vi "VMI_move_wait_PI.vi"(3 "Scan?":bool, 4 "SetV?":bool, 5 "Stage Position 2":refnum<vi>, 6 "Move and Wait?":bool, 7 "Delay Cluster":T1={"System no."=0, "Identification"="", "Device ID out"=0, "Postion / mm"=[], "SN out"="", "Movement Range"=[], "Conn. Axes"=[], "Target Position / mm"=50.0, "Velocity / mm s^-1"=0.15, "Set-up"=FALSE, "Moving"=FALSE, "Step Size / mm "=0.15, "Stage Number"=0, "Polling Time /ms"=0, "Delay Scan?"=FALSE, "Accurate Scan"=FALSE, "CmdMovDelay"=FALSE, "CmdStopDelay"=FALSE, "Delay List"=[["Number", "Target / mm", "Relative Integration Time"]], "Scan Start /mm"=50.0, "Scan End / mm"=80.0, "Scan Velocity / mm s^-1"=0.15, "Delay Scan Time / s"=30.0}, 8 "Error In":errorcluster, 10 "Stop ref":refnum<vi>, 11 "Postion / mm":refnum<vi>) -> (0 "error out":errorcluster)   [LabVIEW 2020]
uses:
  Type defs/PI_delay_settings_alt.ctl
panel:
  out "Stage Position":dbl=50.0
  in  "Stop Button":bool
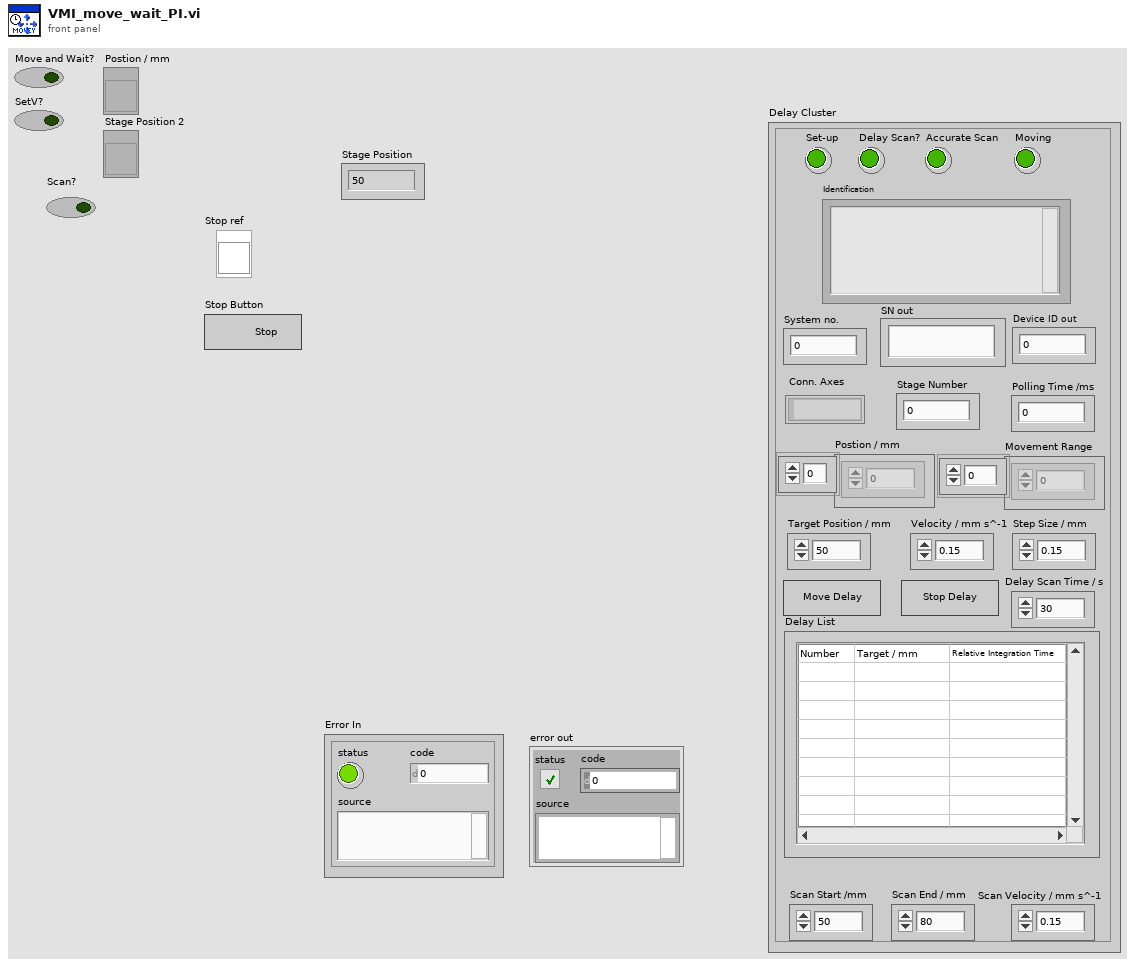
[diagram p1: front panel]
types:
  T1 = typedef "PI_delay_settings_alt.ctl" = cluster{"System no.":i32, "Identification":string, "Device ID out":i32, "Postion / mm":dbl[], "SN out":string, "Movement Range":dbl[], "Conn. Axes":string[], "Target Position / mm":dbl, "Velocity / mm s^-1":dbl, "Set-up":bool, "Moving":bool, "Step Size / mm ":dbl, "Stage Number":i32, "Polling Time /ms":i32, "Delay Scan?":bool, "Accurate Scan":bool, "CmdMovDelay":bool, "CmdStopDelay":bool, "Delay List":string[][], "Scan Start /mm":dbl, "Scan End / mm":dbl, "Scan Velocity / mm s^-1":dbl, "Delay Scan Time / s":dbl}
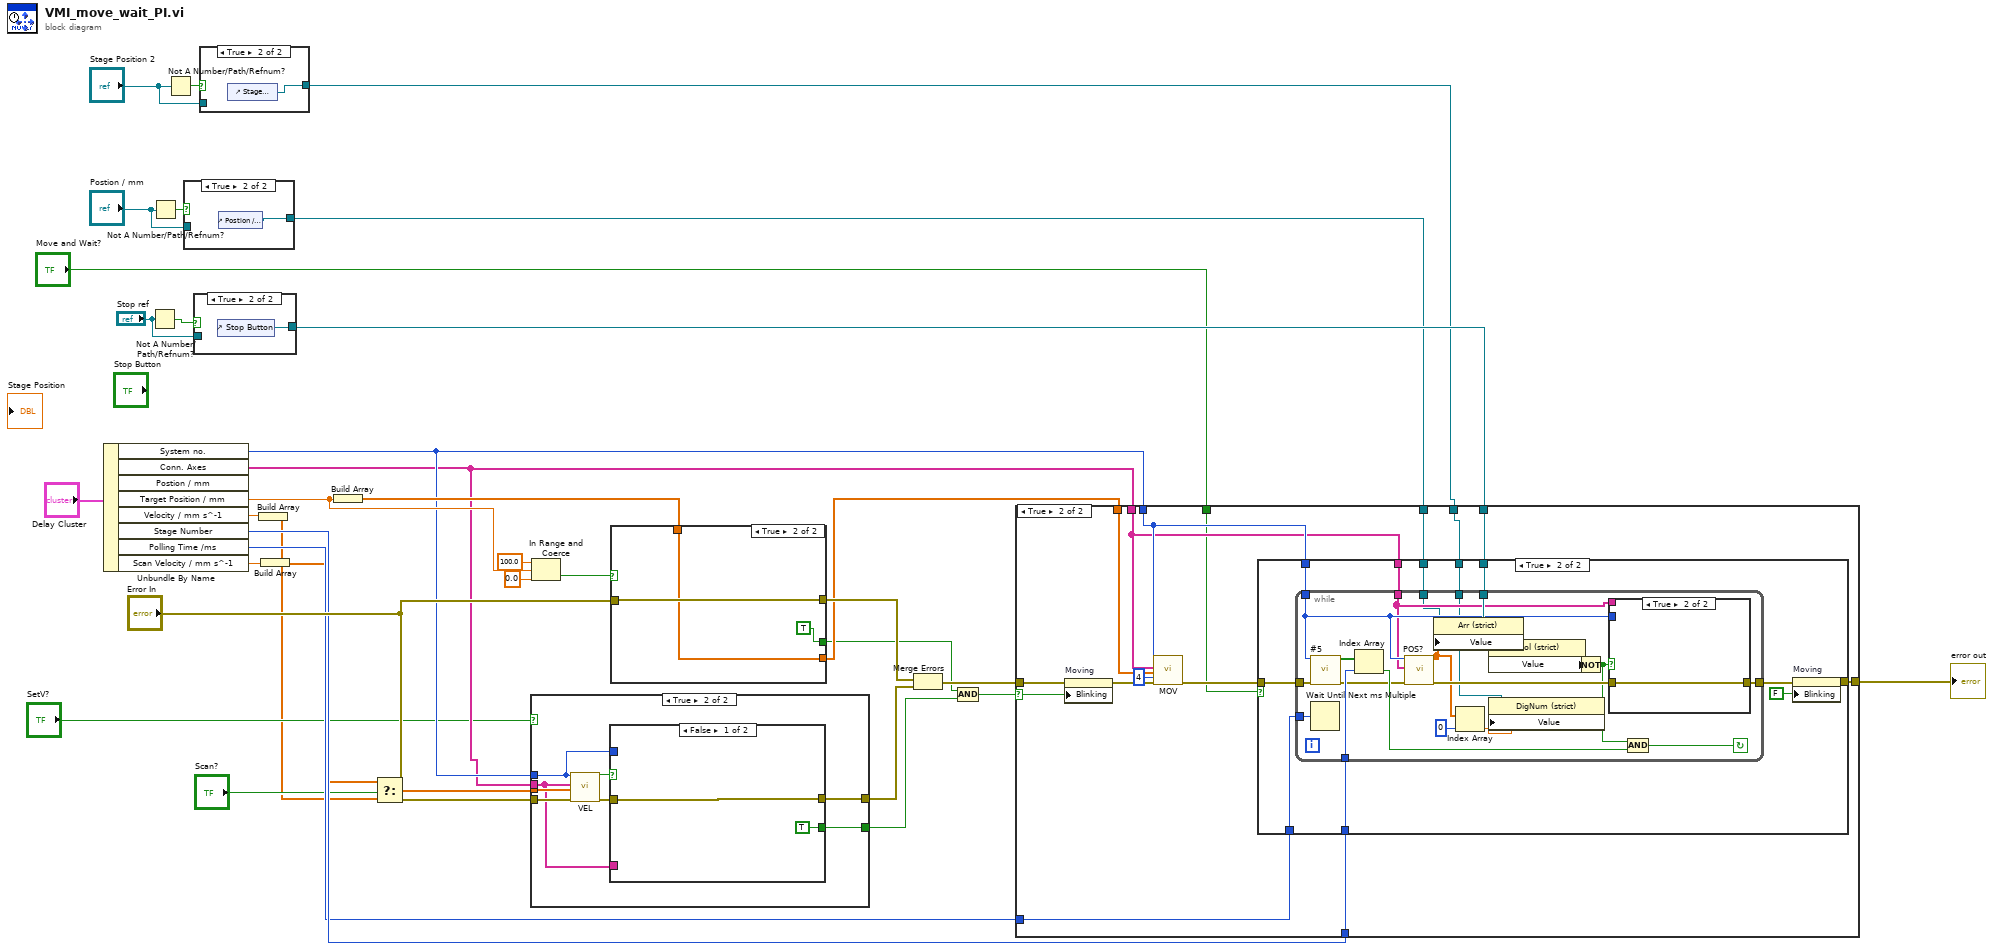
[diagram p0: block diagram]
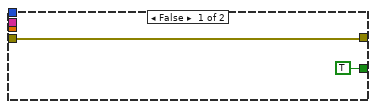
[diagram p3: hidden frame]
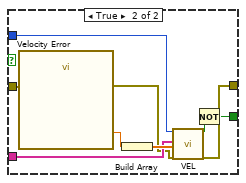
[diagram p4: hidden frame]
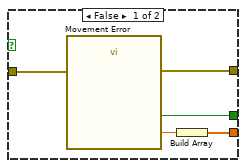
[diagram p7: hidden frame]
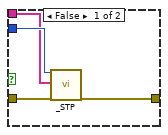
[diagram p10: hidden frame]
diagram:
  n1 = Unbundle By Name("Delay Cluster") -> ("System no."=w18:i32, "Conn. Axes"=w17:string[], "Target Position / mm"=w27:dbl, "Velocity / mm s^-1"=w35:dbl, "Stage Number"=w14:i32, "Polling Time /ms"=w13:i32, "Scan Velocity / mm s^-1"=w8:dbl)  [unwired: 1 out]
  n2 = Not A Number/Path/Refnum?(number/path/refnum="Stop ref") -> (NaN/Path/Refnum?=w21:bool)
  n3 = Not A Number/Path/Refnum?(number/path/refnum="Postion / mm") -> (NaN/Path/Refnum?=w15:bool)
  n4 = Not A Number/Path/Refnum?(number/path/refnum="Stage Position 2") -> (NaN/Path/Refnum?=w3:bool)
  n5 = case shown="True" w15 {
    tunnel: "Postion / mm" -> [w37 _]
    tunnel: [w37 w38] -> w10
    frame False {
    }
    frame True {
      n6 = control-ref of="Postion / mm"() -> (w38:refnum<vi>)
    }
  }
  n7 = case shown="True" w21 {
    tunnel: [w39 w40] -> w19
    tunnel: "Stop ref" -> [w39 _]
    frame False {
    }
    frame True {
      n8 = control-ref of="Stop Button"() -> (w40:refnum<vi>)
    }
  }
  n9 = case shown="True" w3 {
    tunnel: "Stage Position 2" -> [w41 _]
    tunnel: [w41 w42] -> w1
    frame False {
    }
    frame True {
      n10 = control-ref of="Stage Position"() -> (w42:refnum<vi>)
    }
  }
  n11 = Build Array(w35) -> (w5:dbl[])
  n12 = Build Array(w8) -> (w6:dbl[])
  n13 = Build Array(w27) -> (w30:dbl[])
  n14 = Select(t=w6, s="Scan?", f=w5) -> (s? t:f=w4:dbl[])
  n15 = case shown="True" "SetV?" {
    tunnel: w4 -> [_ w52]
    tunnel: "Error In" -> [w44 w49]
    tunnel: [w44 w48] -> w32
    tunnel: [TRUE ("OK") w47] -> w24
    tunnel: w18 -> [_ w46]
    tunnel: w17 -> [_ w45]
    frame False {
    }
    frame True {
      n16 = call "VEL.vi"("System no."=w46, "Axes to set"=w45, "Velocity values"=w52, "error in"=w49) -> ("Controller error"=w51:bool, "error out"=w50:errorcluster)  [unwired: 2 in, 12 out]
      n17 = case shown="False" w51 {
        tunnel: w50 -> [w54 w63]
        tunnel: [w54 w57] -> w48
        tunnel: [TRUE ("OK") w55] -> w47
        tunnel: w46 -> [_ w60]
        tunnel: w45 -> [_ w59]
        frame False {
        }
        frame True {
          n18 = call "Velocity Error"("error in (no error)"=w63) -> ("Velocity"=w62:dbl, "error out"=w58:errorcluster)  [unwired: 16 in, 1 out]
          n19 = Build Array(w62) -> (w61:dbl[])
          n20 = call "VEL.vi"("System no."=w60, "Axes to set"=w59, "Velocity values"=w61, "error in"=w58) -> ("Controller error"=w56:bool, "error out"=w57:errorcluster)  [unwired: 2 in, 12 out]
          n21 = Not(x=w56) -> (.not. x?=w55:bool)
        }
      }
    }
  }
  n22 = In Range and Coerce(upper limit=100.0, x=w27, lower limit=0.0) -> (In Range?=w25:bool)  [unwired: 1 out]
  n23 = case shown="True" w25 {
    tunnel: "Error In" -> [w68 w71]
    tunnel: [w67 w71] -> w33
    tunnel: [w66 TRUE ("OK")] -> w22
    tunnel: [w64 w69] -> w29
    tunnel: w30 -> [_ w69]
    frame False {
      n24 = call "Movement Error"("error in (no error)"=w68) -> ("Target"=w65:dbl, "OK"=w66:bool, "error out"=w67:errorcluster)  [unwired: 16 in]
      n25 = Build Array(w65) -> (w64:dbl[])
    }
    frame True {
    }
  }
  n26 = Merge Errors(w33, w32) -> (w31:errorcluster)
  n27 = And(x=w22, y=w24) -> (x .and. y?=w23:bool)
  n28 = case shown="True" w23 {
    selector: w23 -> [_ w84]
    tunnel: w29 -> [_ w87]
    tunnel: w18 -> [_ w80]
    tunnel: w17 -> [_ w78]
    tunnel: w31 -> [w72 w85]
    tunnel: [w72 w82] -> w16
    tunnel: w14 -> [_ w79]
    tunnel: w19 -> [_ w77]
    tunnel: w13 -> [_ w76]
    tunnel: "Move and Wait?" -> [_ w75]
    tunnel: w10 -> [_ w74]
    tunnel: w1 -> [_ w73]
    frame False {
    }
    frame True {
      n29 = property on="Moving" class="Bool (strict)"(error in=w85, "Blinking"=w84) -> (error out=w83:errorcluster)  [unwired: 1 in, 1 out]
      n30 = call "MOV.vi"("System no."=w80, "Axes to move"=w78, "Position values"=w87, "No.of digits"=i16 4, "error in"=w83) -> ("error out"=w81:errorcluster)  [unwired: 14 out]
      n31 = case shown="True" w75 {
        tunnel: [w88 w99] -> w82
        tunnel: w81 -> [w88 w98]
        tunnel: w80 -> [_ w97]
        tunnel: w79 -> [_ w96]
        tunnel: w78 -> [_ w95]
        tunnel: w77 -> [_ w92]
        tunnel: w76 -> [_ w91]
        tunnel: w74 -> [_ w90]
        tunnel: w73 -> [_ w89]
        frame False {
        }
        frame True {
          n32 = while {
            tunnel: w98 -> [w118]
            tunnel: w97 -> [w106]
            tunnel: w96 -> [w116]
            tunnel: w95 -> [w105]
            tunnel: [w109] -> w94
            tunnel: w91 -> [w113]
            tunnel: w92 -> [w112]
            tunnel: w90 -> [w104]
            tunnel: w89 -> [w100]
            stop <- w108 continue-if-true
            n33 = Wait Until Next ms Multiple(millisecond multiple=w113) -> ()  [unwired: 1 out]
            n34 = call "#5.vi"("System no."=w106, "error in"=w118) -> ("Axis moving?"=w117:bool[], "error out"=w114:errorcluster)  [unwired: 16 in]
            n35 = Index Array(array=w117, index=w116) -> (element=w115:bool)
            n36 = call "POS?.vi"("System no."=w106, "Axes to query"=w105, "error in"=w114) -> ("Position"=w103:dbl[], "error out"=w110:errorcluster)  [unwired: 15 in]
            n37 = property on="Property Node" class="Arr (strict)"(reference=w104, "Value"=w103) -> ()  [unwired: 1 in, 2 out]
            n38 = Index Array(array=w103, index=0) -> (element=w101:dbl)
            n39 = property class="Bool (strict)"(reference=w112) -> ("Value"=w111:bool)  [unwired: 1 in, 2 out]
            n40 = property on="Property Node" class="DigNum (strict)"(reference=w100, "Value"=w101) -> ()  [unwired: 1 in, 2 out]
            n41 = Not(x=w111) -> (.not. x?=w107:bool)
            n42 = case shown="True" w107 {
              tunnel: w110 -> [w122 w123]
              tunnel: [w121 w123] -> w109
              tunnel: w106 -> [w120 _]
              tunnel: w105 -> [w119 _]
              frame False {
                n43 = call "_STP.vi"("System no."=w120, "Affected axes?"=w119, "error in"=w122) -> ("error out"=w121:errorcluster)  [unwired: 16 in]
              }
              frame True {
              }
            }
            n44 = And(x=w107, y=w115) -> (x .and. y?=w108:bool)
          }
          n45 = property on="Moving" class="Bool (strict)"(error in=w94, "Blinking"=FALSE) -> (error out=w99:errorcluster)  [unwired: 1 in, 1 out]
        }
      }
    }
  }
  "error out" <- w16
